vi "Replace Actor if Using PPL.vi"(8 "error in (no error)":errorcluster, 10 "Target":refnum<vi>, 11 "Send VI ref in":refnum<vi>) -> (0 "error out":errorcluster, 3 "Send VI ref out":refnum<vi>)   [LabVIEW 2020, in "Message Maker.lvlib"]
uses:
  Message Maker.lvlib
  <vilib>/Utility/traverseref.llb/TRef TravTarget.ctl
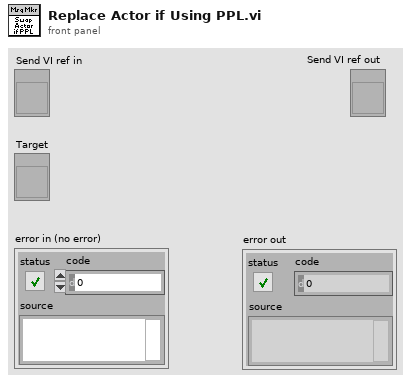
[diagram p1: front panel]
types:
  T1 = typedef "TRef TravTarget.ctl" = enum16{"FP", "BD", "Other"}
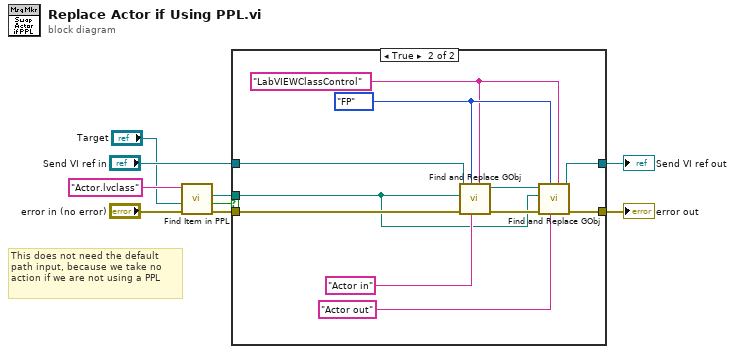
[diagram p0: block diagram]
diagram:
  # "This does not need the default path input, because we take no action if we are not using a PPL"
  n1 = call "Find Item in PPL.vi"("error in (no error)"="error in (no error)", "Target"="Target", "qualified name"="Actor.lvclass") -> ("error out"=w8:errorcluster, "ppl exists?"=w3:bool, "item path out"=w5:path)  [unwired: 6 in]
  n2 = case shown="True" w3 {
    tunnel: w8 -> [w10 w15]
    tunnel: "Send VI ref in" -> [w11 w12]
    tunnel: [w11 w17] -> w6
    tunnel: w5 -> [_ w13]
    tunnel: [w10 w16] -> w2
    frame False {
    }
    frame True {
      w19 = TRef_TravTarget."FP" ("Traverse Target")
      w18 = "LabVIEWClassControl" ("Class Name")
      n3 = call "Find and Replace GObj.vi"("GObj Class Name"=w18, "GObj Label"="Actor in", "Traverse Target"=w19, "error in (no error)"=w15, "Class Path"=w13, "vi reference in"=w12) -> ("error out"=w20:errorcluster, "vi reference out"=w22:refnum<vi>)  [unwired: 3 in, 1 out]
      n4 = call "Find and Replace GObj.vi"("GObj Class Name"=w18, "GObj Label"="Actor out", "Traverse Target"=w19, "error in (no error)"=w20, "Class Path"=w13, "vi reference in"=w22) -> ("error out"=w16:errorcluster, "vi reference out"=w17:refnum<vi>)  [unwired: 3 in, 1 out]
    }
  }
  "Send VI ref out" <- w6
  "error out" <- w2
